vi "Coordinates Conversion.vi"(8 "Coordinates System":enum16{"Cartesian", "Cylindrical", "Spherical"}(ring), 9 "Z in":sgl, 10 "Y in":sgl, 11 "X in":sgl) -> (0 "NaN?":bool, 1 "Z out":sgl, 2 "Y out":sgl, 3 "X out":sgl)   [LabVIEW 2020, in "3D Plot Datatype.lvclass"]
uses:
  3D Plot Datatype.lvclass
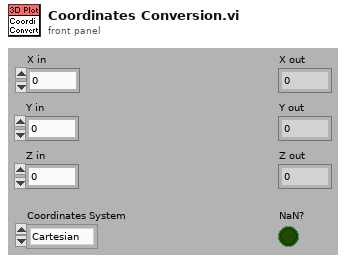
[diagram p1: front panel]
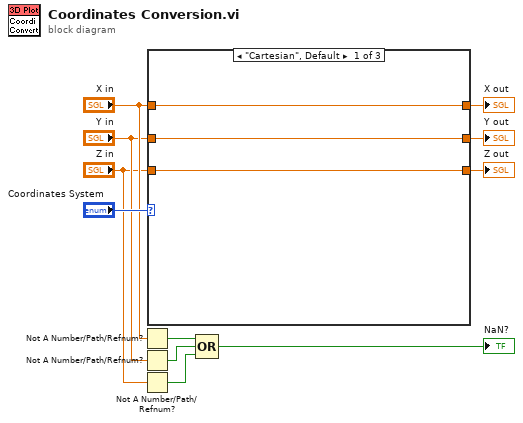
[diagram p0: block diagram]
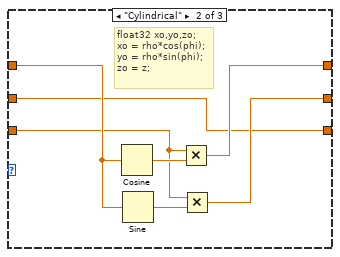
[diagram p2: hidden frame]
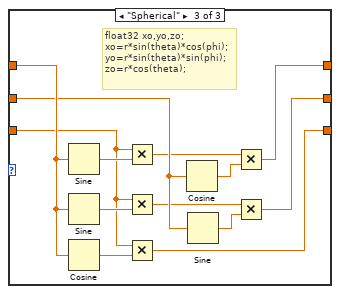
[diagram p3: hidden frame]
diagram:
  n1 = Not A Number/Path/Refnum?(number/path/refnum="X in") -> (NaN/Path/Refnum?=w4:bool)
  n2 = Not A Number/Path/Refnum?(number/path/refnum="Y in") -> (NaN/Path/Refnum?=w3:bool)
  n3 = Not A Number/Path/Refnum?(number/path/refnum="Z in") -> (NaN/Path/Refnum?=w2:bool)
  n4 = case shown="\"Cartesian\", Default" "Coordinates System" {
    tunnel: [w14 w17 w23] -> w10
    tunnel: [w13 w16 w22] -> w9
    tunnel: [w12 w15 w29] -> w8
    tunnel: "X in" -> [w14 w21 w34]
    tunnel: "Z in" -> [w12 w18 w31]
    tunnel: "Y in" -> [w13 w15 w28]
    frame "Cartesian", Default {
    }
    frame "Cylindrical" {
      # "float32 xo,yo,zo;\nxo = rho*cos(phi);\nyo = rho*sin(phi);\nzo = z;"
      n5 = Cosine(x=w21) -> (cos(x)=w20:sgl)
      n6 = Sine(x=w21) -> (sin(x)=w19:sgl)
      n7 = Multiply(x=w18, y=w20) -> (x*y=w17:sgl)
      n8 = Multiply(x=w18, y=w19) -> (x*y=w16:sgl)
    }
    frame "Spherical" {
      # "float32 xo,yo,zo;\nxo=r*sin(theta)*cos(phi);\nyo=r*sin(theta)*sin(phi);\nzo=r*cos(theta);"
      n9 = Sine(x=w34) -> (sin(x)=w33:sgl)
      n10 = Sine(x=w34) -> (sin(x)=w32:sgl)
      n11 = Cosine(x=w34) -> (cos(x)=w30:sgl)
      n12 = Multiply(x=w31, y=w33) -> (x*y=w25:sgl)
      n13 = Multiply(x=w31, y=w32) -> (x*y=w26:sgl)
      n14 = Multiply(x=w31, y=w30) -> (x*y=w29:sgl)
      n15 = Cosine(x=w28) -> (cos(x)=w24:sgl)
      n16 = Sine(x=w28) -> (sin(x)=w27:sgl)
      n17 = Multiply(x=w25, y=w24) -> (x*y=w23:sgl)
      n18 = Multiply(x=w26, y=w27) -> (x*y=w22:sgl)
    }
  }
  "X out" <- w10
  "Y out" <- w9
  "Z out" <- w8
  n19 = Compound Arithmetic op=OR(w4, w3, w2) -> (→"NaN?":bool)
